vi "FranckHertzLogger.vi"() -> ()   [LabVIEW 2014]
uses:
  Typedef_FindPortActions.ctl
  Typedef_TeachLabArduinos.ctl
  Typedef_DataLogger_Actions.ctl
  <vilib>/Utility/file.llb/Write To Spreadsheet File (DBL).vi
panel:
  in  "Time Step (ms)":i32=100 min=5 max=5000 step=1
  out "Elapsed Time (s)":dbl format="%.1f"
  in  "Filename Header":string="Data"
  in  "Maximum Log Time (s)":dbl=60.0
  out "Status":enum16{"Logging", "Stopped"}(ring)=enum."Stopped"
  in  "Logging":cluster{"Start":bool, "Stop":bool}
  out "Last Save's Filename":string
  out "Species":string
  out "Current":dbl format="%.4f"
  out "Scan Voltage (V)":dbl format="%.2f"
  in  "Save Data":bool
  in  "Reset Graph":bool
  out "XY Graph":cluster{dbl[], dbl[]}(graph)
  out "Error Out":errorcluster
  in  "Exit Program":bool
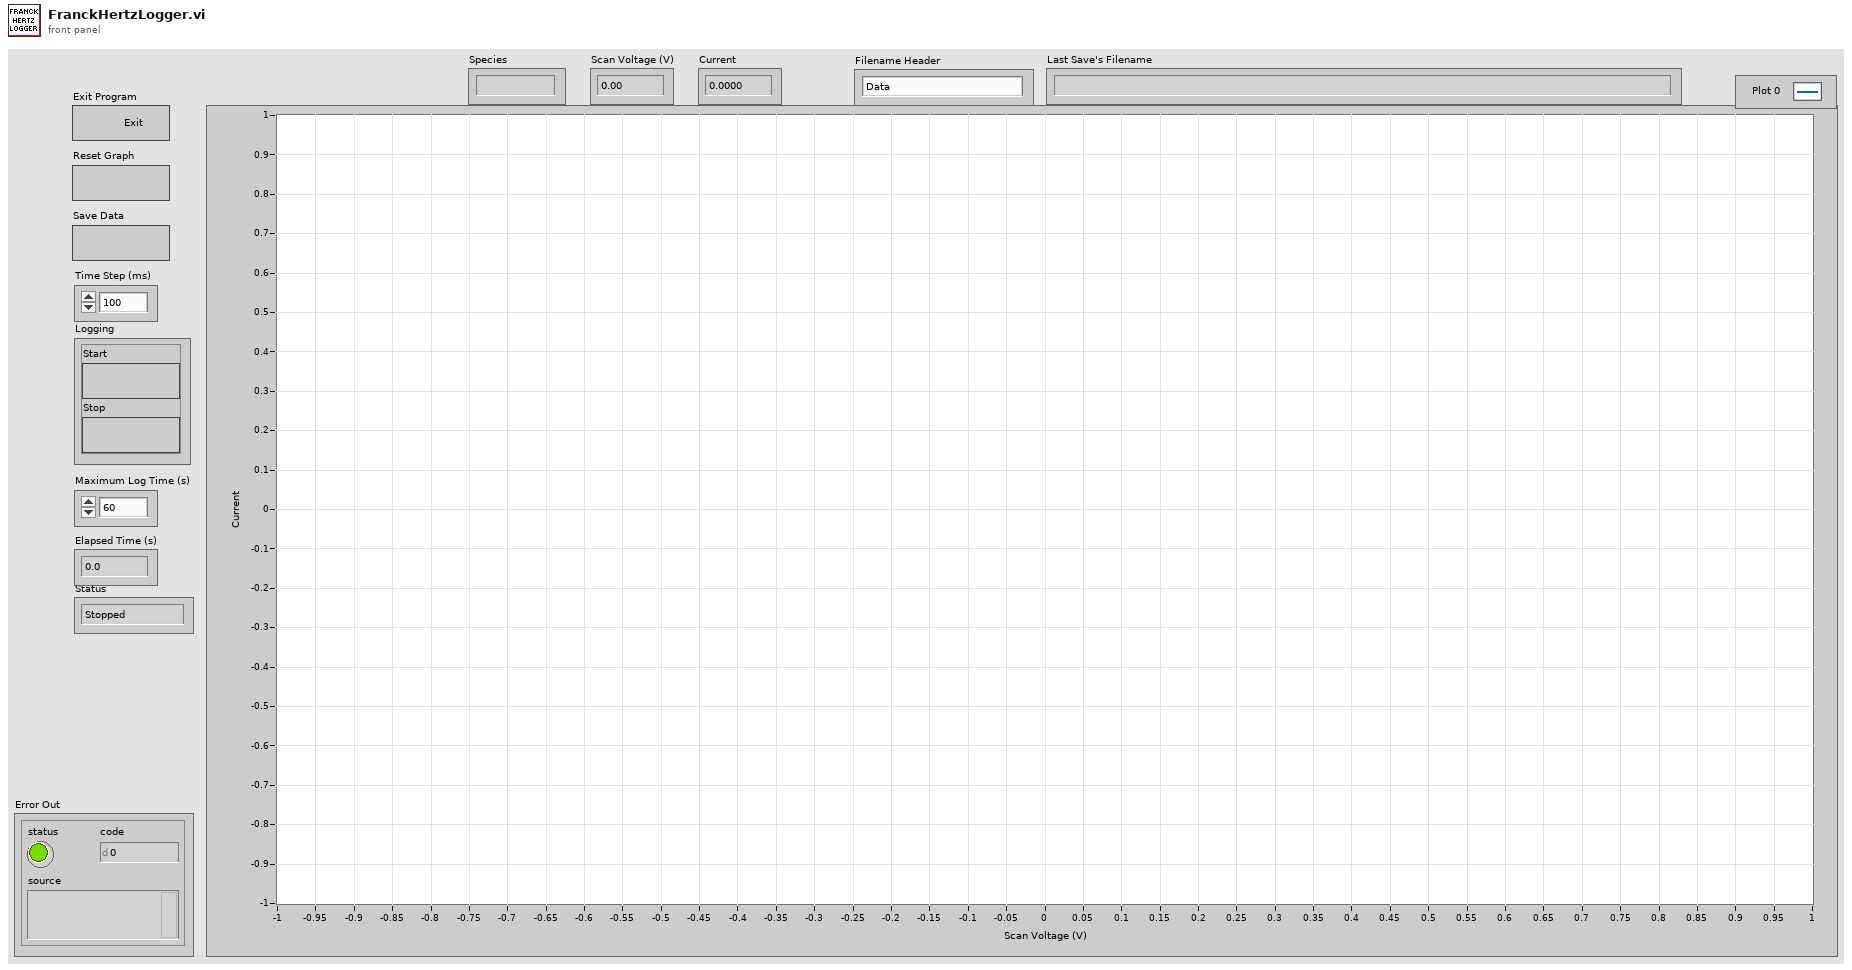
[diagram p1: front panel]
types:
  T1 = typedef "Typedef_FindPortActions.ctl" = enum16{"Reset List", "Find arduinos", "Get COM Port"}
  T2 = typedef "Typedef_TeachLabArduinos.ctl" = enum16{"FH", "AL", "CO"}
  T3 = typedef "Typedef_DataLogger_Actions.ctl" = enum16{"Connect", "Disconnect", "Get Reading", "Set Offset", "Get Offset", "Set Time Step", "Get Time Step", "Save Settings", "Disable Readings", "Enable Readings"}
  T4 = enum32{"invalid app kind", "Development System", "Run Time System", "Student Edition", "Embedded LabVIEW", "Evaluation", "Custom"}
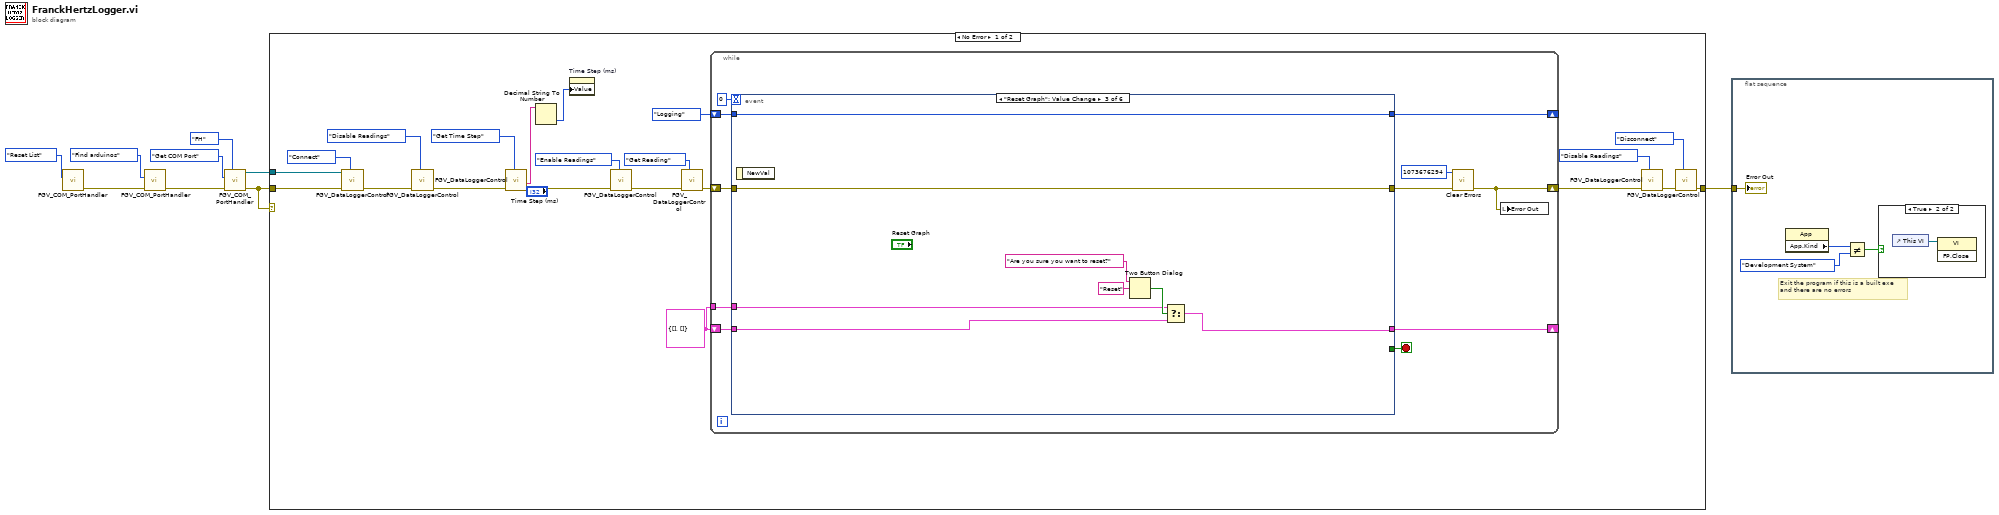
[diagram p0: block diagram]
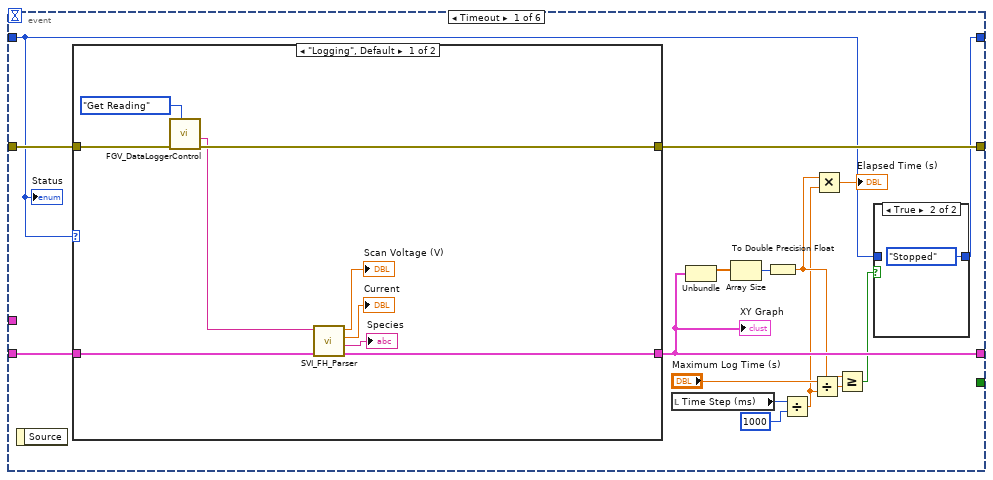
[diagram p3: hidden frame]
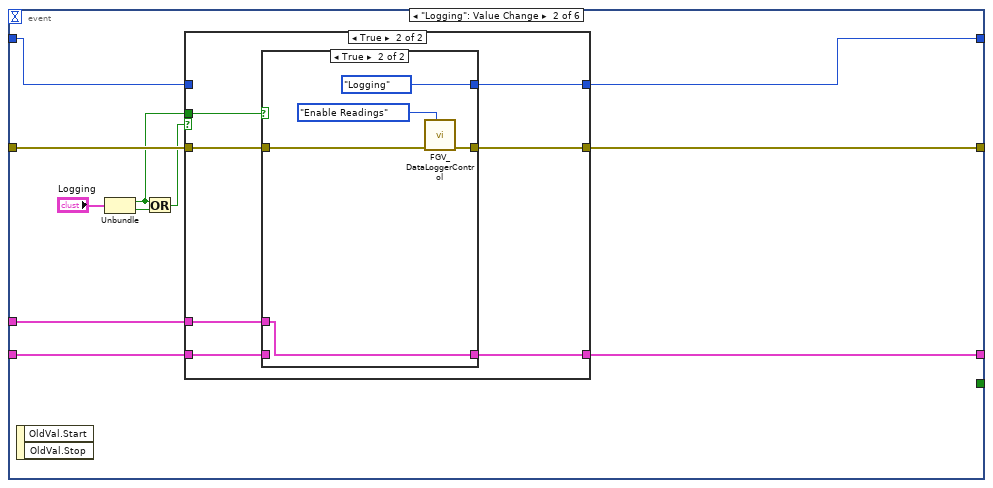
[diagram p6: hidden frame]
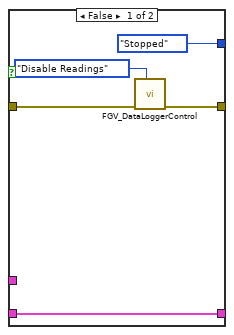
[diagram p8: hidden frame]
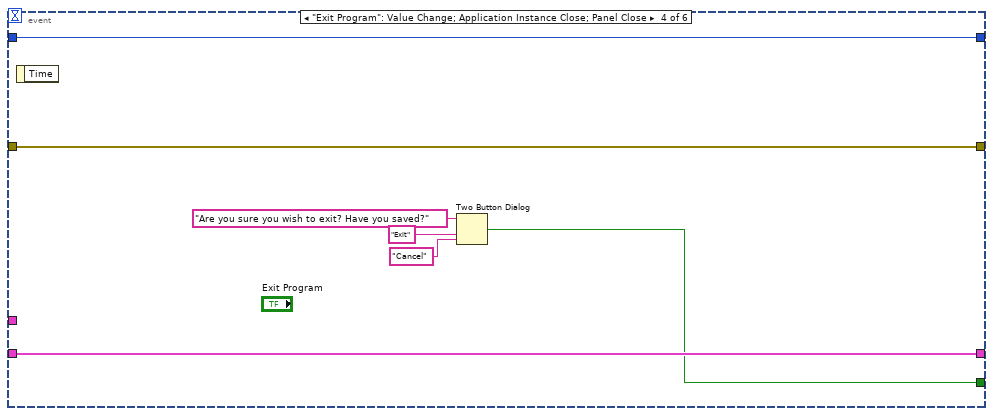
[diagram p9: hidden frame]
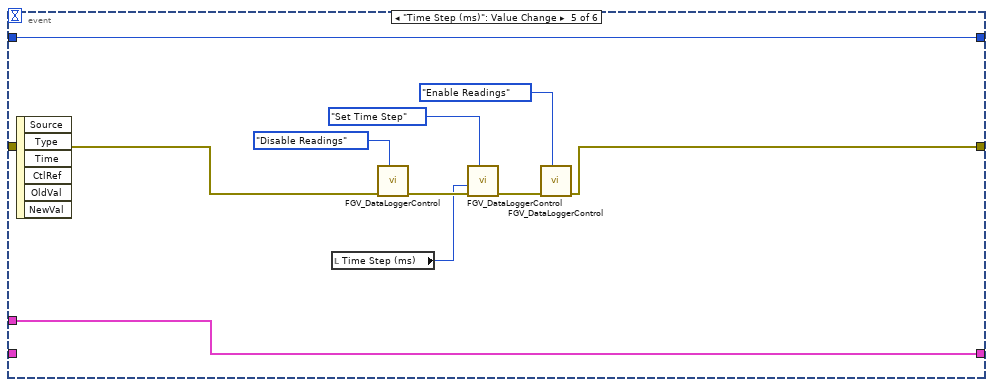
[diagram p10: hidden frame]
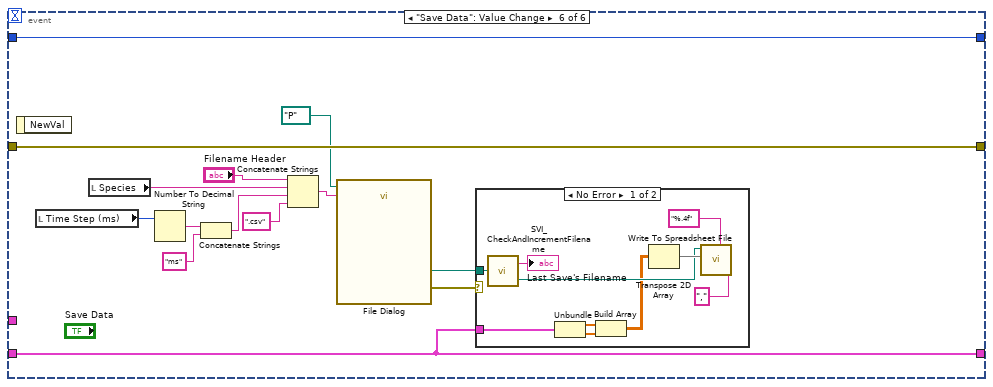
[diagram p11: hidden frame]
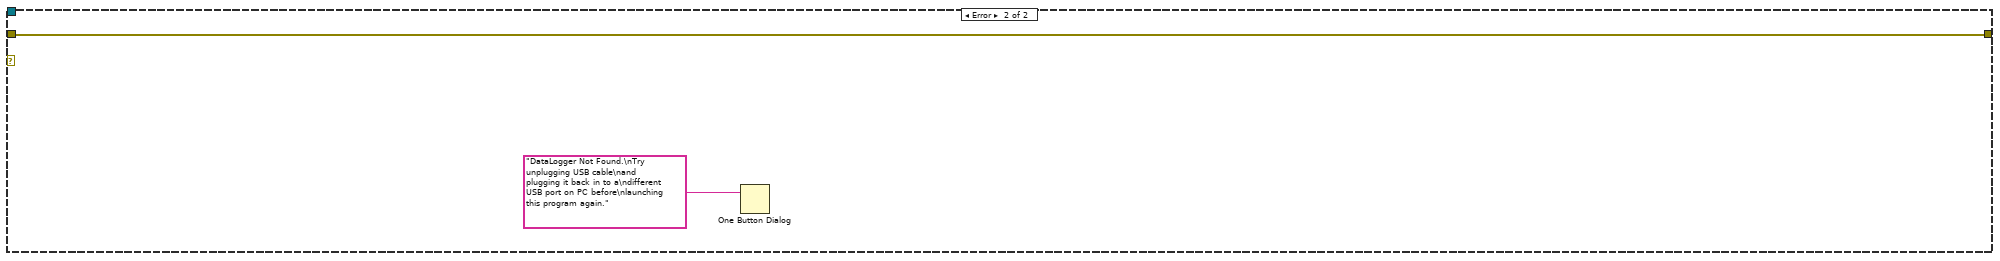
[diagram p13: hidden frame]
diagram:
  n1 = call "FGV_COM_PortHandler.vi"("Action"=Typedef_FindPortActions."Reset List") -> ("Error Out"=w5:errorcluster)  [unwired: 5 in, 2 out]
  n2 = call "FGV_COM_PortHandler.vi"("Error In"=w5, "Action"=Typedef_FindPortActions."Find arduinos") -> ("Error Out"=w9:errorcluster)  [unwired: 4 in, 2 out]
  n3 = call "FGV_COM_PortHandler.vi"("Device"=Typedef_TeachLabArduinos."FH", "Error In"=w9, "Action"=Typedef_FindPortActions."Get COM Port") -> ("Error Out"=w2:errorcluster, "COM Port"=w3:refnum<visa-resource-name>)  [unwired: 3 in, 1 out]
  n4 = case shown="No Error" w2 {
    tunnel: w2 -> [w29 w152]
    tunnel: w3 -> [w28 _]
    tunnel: [w25 w152] -> w1
    frame No Error {
      w14 = cluster{dbl[], dbl[]} {[], []}
      n5 = call "FGV_DataLoggerControl.vi"("Actions"=Typedef_DataLogger_Actions."Connect", "Error In"=w29, "VISA Refnum in"=w28) -> ("Error Out"=w21:errorcluster)  [unwired: 6 in, 2 out]
      n6 = call "FGV_DataLoggerControl.vi"("Actions"=Typedef_DataLogger_Actions."Disable Readings", "Error In"=w21) -> ("Error Out"=w20:errorcluster)  [unwired: 7 in, 2 out]
      n7 = call "FGV_DataLoggerControl.vi"("Actions"=Typedef_DataLogger_Actions."Get Time Step", "Error In"=w20) -> ("Error Out"=w18:errorcluster, "read buffer"=w24:string)  [unwired: 7 in, 1 out]
      n8 = Decimal String To Number(string=w24) -> (number=w23:i32)  [unwired: 2 in, 1 out]
      n9 = property on="Time Step (ms)" class="DigNum (strict)"("Value"=w23) -> ()  [unwired: 2 in, 2 out]
      n10 = call "FGV_DataLoggerControl.vi"("Actions"=Typedef_DataLogger_Actions."Enable Readings", "Error In"=w18) -> ("Error Out"=w10:errorcluster)  [unwired: 7 in, 2 out]
      n11 = call "FGV_DataLoggerControl.vi"("Actions"=Typedef_DataLogger_Actions."Get Reading", "Error In"=w10) -> ("Error Out"=w11:errorcluster)  [unwired: 7 in, 2 out]
      n12 = while {
        shift-right: [w38] -> _
        shift-left: w14 -> [w37]
        tunnel: w14 -> [w36]
        shift-right: [w34] -> _
        shift-left: enum16{"Logging", "Stopped"}."Logging" ("Status") -> [w35]
        shift-right: [w32] -> w16
        shift-left: w11 -> [w41]
        stop <- w40 stop-if-true
        n13 = event shown="[2] \"Reset Graph\": Value Change" {
          selector: _ -> [_ _ _ _ _ _]
          dyn-events: _ -> [_ _ _ _ _ _]
          timeout: 0 -> [_ _ _ _ _ _]
          tunnel: w41 -> [w57 w79 w109 w115 w119 w140]
          tunnel: [w56 w78 w109 w115 w120 w140] -> w31
          tunnel: [_ _ _ w111 _ _] -> w40
          tunnel: [w53 w72 w104 w116 w118 w139] -> w38
          tunnel: w37 -> [w55 w73 w102 w116 _ w139]
          tunnel: w36 -> [_ w71 w103 _ w118 _]
          tunnel: [w46 w81 w108 w110 w117 w130] -> w34
          tunnel: w35 -> [w45 w80 w108 w110 w117 w130]
          event Timeout {
            n14 = event-data() -> ()  [unwired: 1 in, 1 out]
            n15 = case shown="\"Logging\", Default" w45 {
              tunnel: w57 -> [w68 w69]
              tunnel: [w67 w69] -> w56
              tunnel: [w64 w70] -> w53
              tunnel: w55 -> [w63 w70]
              frame "Logging", Default {
                n16 = call "FGV_DataLoggerControl.vi"("Actions"=Typedef_DataLogger_Actions."Get Reading", "Error In"=w68) -> ("Error Out"=w67:errorcluster, "read buffer"=w65:string)  [unwired: 7 in, 1 out]
                n17 = call "SVI_FH_Parser.vi"("Cluster in"=w63, "read buffer"=w65) -> ("Cluster out"=w64:cluster{"Array":dbl[], "Array":dbl[]}, "Species"=→"Species":string, "Current"=→"Current":dbl, "Scan Voltage (V)"=→"Scan Voltage (V)":dbl)  [unwired: 2 in]
              }
              frame "Stopped" {
              }
            }
            "XY Graph" <- w53
            n18 = local read "Time Step (ms)"() -> (w52:i32)
            n19 = Unbundle(w53) -> ("Array"=w54:dbl[])  [unwired: 1 out]
            n20 = Array Size(array=w54) -> (size(s)=w48:i32)
            n21 = To Double Precision Float(number=w48) -> (double precision float=w44:dbl)
            n22 = Divide(x=w52, y=1000) -> (x/y=w43:dbl)
            n23 = Divide(x="Maximum Log Time (s)", y=w43) -> (x/y=w49:dbl)
            n24 = Multiply(x=w44, y=w43) -> (x*y=→"Elapsed Time (s)":dbl)
            n25 = Greater Or Equal?(x=w44, y=w49) -> (x >= y?=w47:bool)
            n26 = case shown="True" w47 {
              tunnel: [w58 enum16{"Logging", "Stopped"}."Stopped" ("Status")] -> w46
              tunnel: w45 -> [w58 _]
              frame False {
              }
              frame True {
              }
            }
            "Status" <- w45
          }
          event "Logging": Value Change {
            n27 = event-data() -> ()  [unwired: 1 in, 2 out]
            n28 = Unbundle("Logging") -> ("Start"=w74:bool, "Stop"=w76:bool)
            n29 = Or(x=w74, y=w76) -> (x .or. y?=w75:bool)
            n30 = case shown="True" w75 {
              tunnel: [w84 w91] -> w81
              tunnel: w80 -> [w84 _]
              tunnel: w79 -> [w83 w90]
              tunnel: [w83 w89] -> w78
              tunnel: w74 -> [_ w88]
              tunnel: w73 -> [w82 w87]
              tunnel: [w82 w86] -> w72
              tunnel: w71 -> [_ w85]
              frame False {
              }
              frame True {
                n31 = case shown="True" w88 {
                  tunnel: [enum16{"Logging", "Stopped"}."Stopped" ("Status") enum16{"Logging", "Stopped"}."Logging" ("Status")] -> w91
                  tunnel: w90 -> [w93 w99]
                  tunnel: [w94 w98] -> w89
                  tunnel: w87 -> [w92 _]
                  tunnel: [w92 w97] -> w86
                  tunnel: w85 -> [_ w97]
                  frame False {
                    n32 = call "FGV_DataLoggerControl.vi"("Actions"=Typedef_DataLogger_Actions."Disable Readings", "Error In"=w93) -> ("Error Out"=w94:errorcluster)  [unwired: 7 in, 2 out]
                  }
                  frame True {
                    n33 = call "FGV_DataLoggerControl.vi"("Actions"=Typedef_DataLogger_Actions."Enable Readings", "Error In"=w99) -> ("Error Out"=w98:errorcluster)  [unwired: 7 in, 2 out]
                  }
                }
              }
            }
          }
          event "Reset Graph": Value Change {
            n34 = event-data() -> ()  [unwired: 1 in, 1 out]
            n35 = Two Button Dialog(message="Are you sure you want to reset?", 2:"Reset" ("T button name (\"OK\")")) -> (T button?=w106:bool)  [unwired: 1 in]
            n36 = Select(t=w103, s=w106, f=w102) -> (s? t:f=w104:cluster{dbl[], dbl[]})
          }
          event "Exit Program": Value Change; Application Instance Close; Panel Close {
            n37 = event-data() -> ()  [unwired: 1 in, 1 out]
            n38 = Two Button Dialog(message="Are you sure you wish to exit? Have you saved?", 1:"Cancel" ("F button name (\"Cancel\")"), 2:"Exit" ("T button name (\"OK\")")) -> (T button?=w111:bool)
          }
          event "Time Step (ms)": Value Change {
            n39 = event-data() -> ()  [unwired: 1 in, 6 out]
            n40 = local read "Time Step (ms)"() -> (w121:i32)
            n41 = call "FGV_DataLoggerControl.vi"("Actions"=Typedef_DataLogger_Actions."Disable Readings", "Error In"=w119) -> ("Error Out"=w124:errorcluster)  [unwired: 7 in, 2 out]
            n42 = call "FGV_DataLoggerControl.vi"("Actions"=Typedef_DataLogger_Actions."Set Time Step", "Error In"=w124, "Value"=w121) -> ("Error Out"=w122:errorcluster)  [unwired: 6 in, 2 out]
            n43 = call "FGV_DataLoggerControl.vi"("Actions"=Typedef_DataLogger_Actions."Enable Readings", "Error In"=w122) -> ("Error Out"=w120:errorcluster)  [unwired: 7 in, 2 out]
          }
          event "Save Data": Value Change {
            n44 = event-data() -> ()  [unwired: 1 in, 1 out]
            n45 = local read "Time Step (ms)"() -> (w131:i32)
            n46 = local read "Species"() -> (w137:string)
            n47 = Number To Decimal String(number=w131) -> (decimal integer string=w132:string)  [unwired: 1 in]
            n48 = Concatenate Strings(w132, "ms" ("string")) -> (w134:string)
            n49 = Concatenate Strings("Filename Header", w137, w134, ".csv" ("default name")) -> (w136:string)
            n50 = call "File Dialog"("start path"=path "P:/", "default name"=w136) -> ("selected path"=w138:path, "error out"=w127:errorcluster)  [unwired: 10 in, 2 out]
            n51 = case shown="No Error" w127 {
              tunnel: w139 -> [w150 _]
              tunnel: w138 -> [w146 _]
              frame No Error {
                n52 = call "SVI_CheckAndIncrementFilename.vi"("selected path"=w146) -> ("Filename"=→"Last Save's Filename":string, "File Path"=w143:path)
                n53 = Unbundle(w150) -> (w148:dbl[], w149:dbl[])
                n54 = Build Array(w148, w149) -> (w142:dbl[][])
                n55 = Transpose 2D Array(2D array=w142) -> (transposed array=w144:dbl[][])
                n56 = call-poly <vilib>:"Write To Spreadsheet File.vi"("delimiter (\\t)"="," ("delimiter (\\t)"), "format (%.3f)"="%.4f", "2D data"=w144, "file path (dialog if empty)"=w143) -> ()  [unwired: 4 in, 1 out]
              }
              frame Error {
              }
            }
          }
        }
        n57 = call <vilib>:"Clear Errors.vi"("error in (no error)"=w31, "specific error code to clear (0: all)"=1073676294) -> ("error out"=w32:errorcluster)  [unwired: 4 in, 1 out]
        n58 = local write "Error Out"(w32) -> ()
      }
      n59 = call "FGV_DataLoggerControl.vi"("Actions"=Typedef_DataLogger_Actions."Disable Readings", "Error In"=w16) -> ("Error Out"=w15:errorcluster)  [unwired: 7 in, 2 out]
      n60 = call "FGV_DataLoggerControl.vi"("Actions"=Typedef_DataLogger_Actions."Disconnect", "Error In"=w15) -> ("Error Out"=w25:errorcluster)  [unwired: 7 in, 2 out]
    }
    frame Error {
      n61 = One Button Dialog(message="DataLogger Not Found.\nTry unplugging USB cable\nand plugging it back in to a\ndifferent USB port on PC before\nlaunching this program again.") -> ()  [unwired: 1 in, 1 out]
    }
  }
  n62 = flat-sequence {
    tunnel: w1 -> [w154]
    frame #0 {
      # "Exit the program if this is a built exe\nand there are no errors"
      n63 = property class="App"() -> ("App.Kind"=w155:T4)  [unwired: 2 in, 2 out]
      n64 = Not Equal?(x=w155, y=T4."Development System" ("Application:Kind 2")) -> (x != y?=w153:bool)
      n65 = case shown="True" w153 {
        frame False {
        }
        frame True {
          n66 = control-ref of="This VI"() -> (w157:refnum<vi>)
          n67 = invoke class="VI" method="FP.Close"(reference=w157) -> ()  [unwired: 2 in, 3 out]
        }
      }
      "Error Out" <- w154
    }
  }
